vi "Read Path.vi"(8 "error in (no error)":errorcluster, 11 "Txt in":refnum<class "Txt.lvclass">) -> (0 "error out":errorcluster, 2 "Path":path, 3 "Txt out":refnum<class "Txt.lvclass">)   [LabVIEW 2020, in "Txt.lvlib" / "Txt.lvclass"]
uses:
  Txt.lvclass
  Txt.lvclass/Txt.ctl
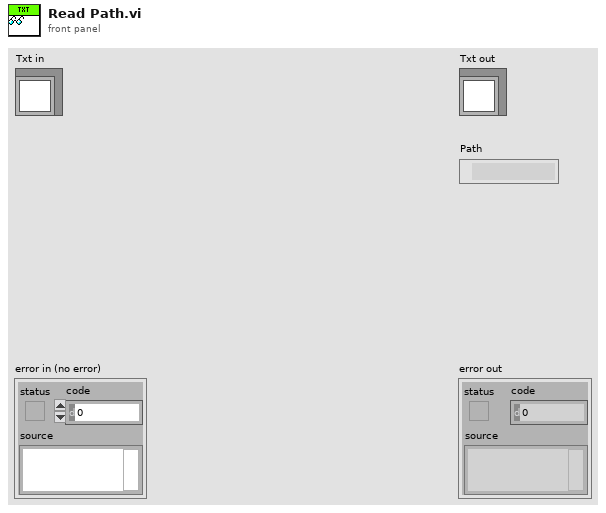
[diagram p1: front panel]
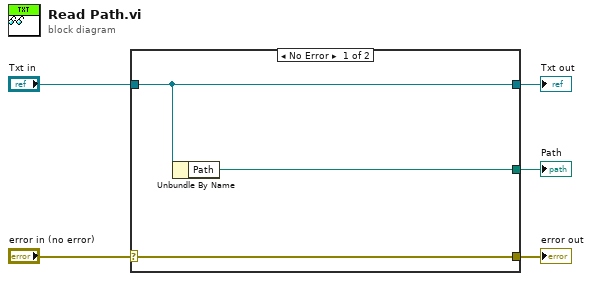
[diagram p0: block diagram]
diagram:
  n1 = case shown="No Error" "error in (no error)" {
    selector: "error in (no error)" -> [w8 w9]
    tunnel: [w8 w9] -> w4
    tunnel: [w7 w10] -> w2
    tunnel: "Txt in" -> [w7 w10]
    tunnel: [w6 _] -> w1
    frame No Error {
      n2 = Unbundle By Name(w7) -> ("Path"=w6:path)
    }
    frame Error {
    }
  }
  "error out" <- w4
  "Txt out" <- w2
  "Path" <- w1
